vi "Process Buttons.vi"(11 "NXT":T1={"Hardware"="NXT", "Flattened String"=""}) -> (3 "NXT":T1={"Hardware"="NXT", "Flattened String"=""})   [LabVIEW 2010, in "FTC.lvlib" / "Remote Interface.lvlib"]
uses:
  Remote Interface.lvlib
  <vilib>/NXT/Subs/LVHSConnector.ctl
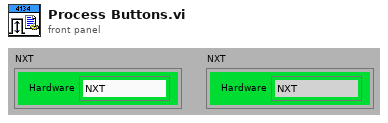
[diagram p1: front panel]
types:
  T1 = typedef "LVHSConnector.ctl" = cluster{"Hardware":string, "Flattened String":string}
  T2 = typedef "CRef.lvlib/I32 CReference.ctl" = cluster{"Generic CRef Address":u16, "Type":enum8{"Null", "Boolean", "U8", "I8", "U16", "I16", "U32", "I32", "U64", "I64", "Single", "Double", "Extended", "CSG", "CDB", "CXT", "Invalid Def", "U8(Def)", "I8(Def)", "U16(Def)", "I16(Def)", "U32(Def)", "I32(Def)"}}
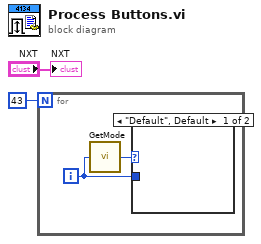
[diagram p0: block diagram]
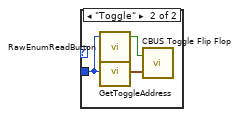
[diagram p2: hidden frame]
diagram:
  n1 = for {
    N: 43 -> [_]
    i -> [w3]
    n2 = call "GetMode.vi"("Button"=w3) -> ("Mode"=w4:enum16{"Default", "Toggle"})
    n3 = case shown="\"Default\", Default" w4 {
      tunnel: w3 -> [_ w5]
      frame "Default", Default {
      }
      frame "Toggle" {
        n4 = call "RawEnumReadButton.vi"("Button"=w5) -> ("Pressed?"=w6:bool)  [unwired: 4 in]
        n5 = call "GetToggleAddress.vi"("Button"=w5) -> ("Address"=w7:T2)
        n6 = call "CBUS Toggle Flip Flop.vi"("CBUS I32 Address"=w7, "Input"=w6) -> ()  [unwired: 1 out]
      }
    }
  }
  "NXT" <- "NXT"
